vi "indexToPoint.vi"(0 "object in":refnum<class "Evaluator.lvclass">, 1 "row":dbl, 2 "col":dbl, 3 "matrixSize":i32[](array[numeric]), 4 "Field":refnum<class "Field.lvclass">, 5 "error in (no error)":errorcluster) -> (14 "object out":refnum<class "Evaluator.lvclass">, 16 "point":dbl[](array[numeric]), 19 "error out":errorcluster)   [LabVIEW 2023, in "Evaluator.lvclass"]
uses:
  Evaluator.lvclass
  Field_class/Field.lvclass
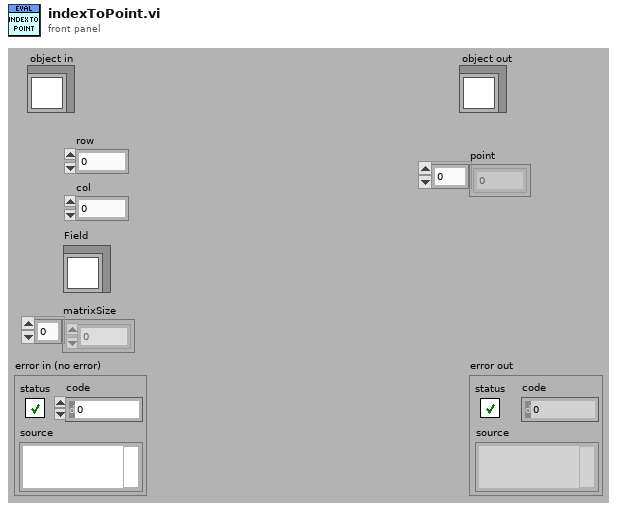
[diagram p1: front panel]
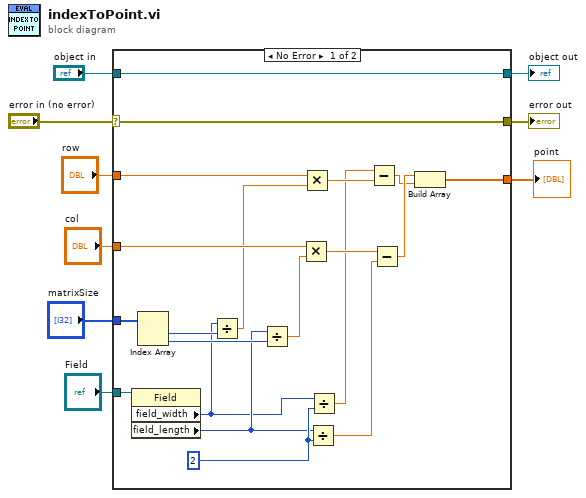
[diagram p0: block diagram]
diagram:
  n1 = case shown="No Error" "error in (no error)" {
    selector: "error in (no error)" -> [w28 w31]
    tunnel: [w28 w31] -> w8
    tunnel: [w29 w30] -> w6
    tunnel: "object in" -> [w29 w30]
    tunnel: "Field" -> [w27 _]
    tunnel: "row" -> [w24 _]
    tunnel: "col" -> [w22 _]
    tunnel: [w10 _] -> w2
    tunnel: "matrixSize" -> [w25 _]
    frame No Error {
      w26 = 2 ("y")
      n2 = property class="Field"(reference=w27) -> ("field_width"=w13:i32, "field_length"=w14:i32)  [unwired: 1 in, 2 out]
      n3 = Index Array(array=w25) -> (element #1=w18:i32, element #2=w17:i32)  [unwired: 2 in]
      n4 = Divide(x=w13, y=w18) -> (x/y=w20:dbl)
      n5 = Divide(x=w14, y=w17) -> (x/y=w19:dbl)
      n6 = Multiply(x=w22, y=w19) -> (x*y=w21:dbl)
      n7 = Multiply(x=w24, y=w20) -> (x*y=w23:dbl)
      n8 = Divide(x=w14, y=w26) -> (x/y=w15:dbl)
      n9 = Divide(x=w13, y=w26) -> (x/y=w16:dbl)
      n10 = Subtract(x=w16, y=w23) -> (x-y=w11:dbl)
      n11 = Subtract(x=w21, y=w15) -> (x-y=w12:dbl)
      n12 = Build Array(w12, w11) -> (w10:dbl[])
    }
    frame Error {
    }
  }
  "error out" <- w8
  "object out" <- w6
  "point" <- w2
